vi "Rotate Front Panel Knob Right.vi"(8 "error in (no error)":errorcluster, 11 "VISA resource name":refnum<visa-resource-name>) -> (0 "error out":errorcluster, 3 "VISA resource name out":refnum<visa-resource-name>)   [LabVIEW 2013, in "SRS SR400.lvlib"]
doc: "<B>RR</B>\n\nRotate front panel knob right (CW or UP) 1 step."
uses:
  <instrlib>/SRS SR400/SRS SR400.lvlib
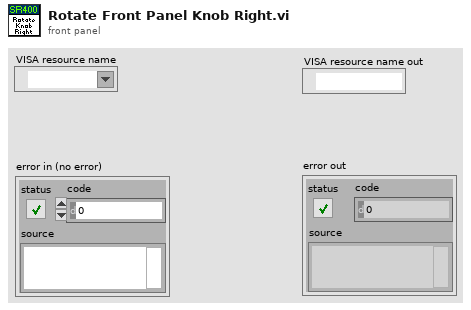
[diagram p1: front panel]
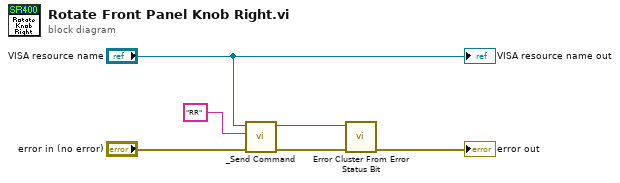
[diagram p0: block diagram]
diagram:
  n1 = call <instrlib>:"_Send Command.vi"("error in (no error)"="error in (no error)", "Command"="RR", "VISA resource name"="VISA resource name") -> ("error out"=w5:errorcluster, "VISA resource name out"=w2:refnum<visa-resource-name>)  [unwired: 6 in, 1 out]
  n2 = call <instrlib>:"Error Cluster From Error Status Bit.vi"("error in (no error)"=w5, "VISA resource name"=w2) -> ("error out"=→"error out":errorcluster)  [unwired: 8 in, 1 out]
  "VISA resource name out" <- "VISA resource name"
